vi "addSimulator.vi"(8 "error in (no error)":errorcluster, 10 "IDevice in":refnum<class "IDevice.lvclass">, 11 "IInstance in":refnum<class "IInstance.lvclass">) -> (0 "error out":errorcluster, 2 "IDevice out":refnum<class "IDevice.lvclass">, 3 "IInstance out":refnum<class "IInstance.lvclass">)   [LabVIEW 2022 SP3, in "openDAQ.lvlib" / "daqUtils.lvlib"]
uses:
  daqUtils.lvlib
  IInstance/IInstance.lvclass
  IDevice/IDevice.lvclass
  IDeviceInfo/IDeviceInfo.lvclass
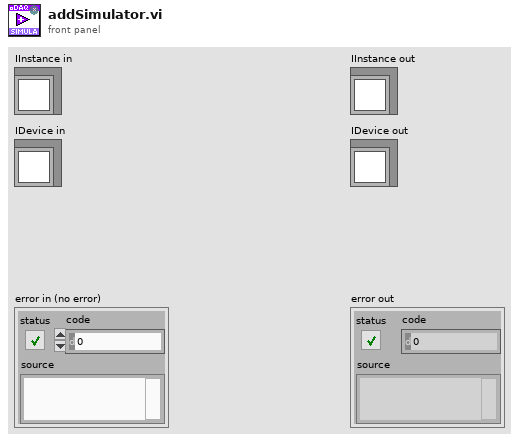
[diagram p1: front panel]
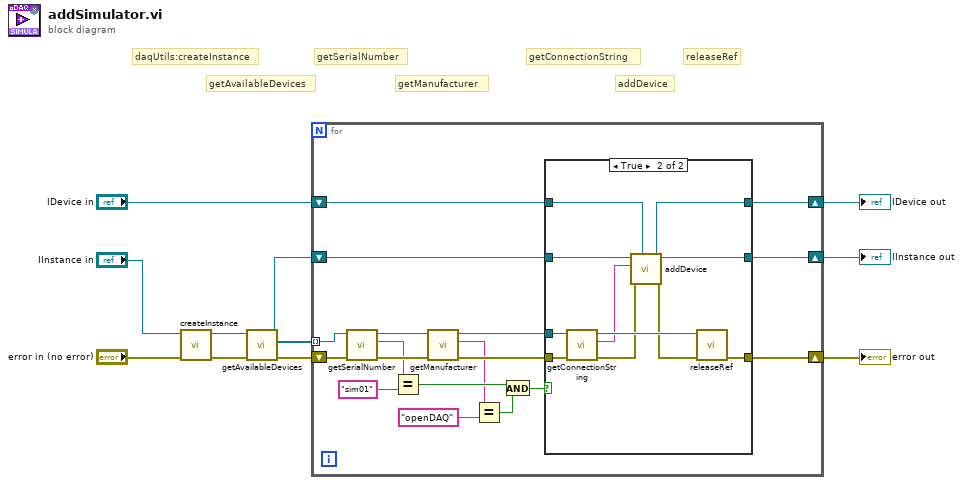
[diagram p0: block diagram]
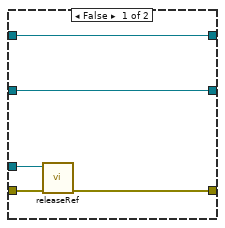
[diagram p2: hidden frame]
diagram:
  # "releaseRef"
  # "addDevice"
  # "getConnectionString"
  # "getManufacturer"
  # "getSerialNumber"
  # "getAvailableDevices"
  # "daqUtils:createInstance"
  n1 = call "createInstance.vi"("error in (no error)"="error in (no error)", "IInstance in"="IInstance in") -> ("error out"=w4:errorcluster, "IInstance out"=w3:refnum<class "IInstance.lvclass">)  [unwired: 8 in]
  n2 = call "getAvailableDevices.vi"("error in (no error)"=w4, "IDevice in"=w3) -> ("error out"=w6:errorcluster, "availableDeviceInfo out"=w5:refnum<class "IDeviceInfo.lvclass">[], "IDevice out"=w7:refnum<class "IInstance.lvclass">)  [unwired: 7 in]
  n3 = for {
    tunnel: w5 -> [w29] mode=indexing
    shift-right: [w20] -> w9
    shift-left: w6 -> [w28]
    shift-right: [w17] -> w10
    shift-left: "IDevice in" -> [w18]
    shift-right: [w16] -> w11
    shift-left: w7 -> [w19]
    n4 = call "getSerialNumber.vi"("error in (no error)"=w28, "IDeviceInfo in"=w29) -> ("error out"=w27:errorcluster, "SerialNumber out"=w15:string, "IDeviceInfo out"=w13:refnum<class "IDeviceInfo.lvclass">)  [unwired: 7 in]
    n5 = Equal?(x=w15, y="sim01") -> (x = y?=w24:bool)
    n6 = call "getManufacturer.vi"("error in (no error)"=w27, "IDeviceInfo in"=w13) -> ("error out"=w21:errorcluster, "Manufacturer out"=w14:string, "IDeviceInfo out"=w12:refnum<class "IDeviceInfo.lvclass">)  [unwired: 7 in]
    n7 = Equal?(x=w14, y="openDAQ") -> (x = y?=w23:bool)
    n8 = And(x=w24, y=w23) -> (x .and. y?=w22:bool)
    n9 = case shown="True" w22 {
      tunnel: w12 -> [w34 w45]
      tunnel: w21 -> [w33 w44]
      tunnel: [w32 w42] -> w20
      tunnel: w19 -> [w30 w41]
      tunnel: w18 -> [w31 w37]
      tunnel: [w31 w35] -> w17
      tunnel: [w30 w36] -> w16
      frame False {
        n10 = call-dynamic "releaseRef.vi"("error in (no error)"=w33, "IBaseObject in"=w34) -> ("error out"=w32:errorcluster)  [unwired: 9 in]
      }
      frame True {
        n11 = call "getConnectionString.vi"("error in (no error)"=w44, "IDeviceInfo in"=w45) -> ("error out"=w40:errorcluster, "ConntectionString out"=w38:string, "IDeviceInfo out"=w43:refnum<class "IDeviceInfo.lvclass">)  [unwired: 7 in]
        n12 = call "addDevice.vi"("ConnectedDevice In"=w37, "error in (no error)"=w40, "ConnectionString in"=w38, "IDevice in"=w41) -> ("error out"=w39:errorcluster, "ConnectedDevice out"=w35:refnum<class "IDevice.lvclass">, "IDevice out"=w36:refnum<class "IInstance.lvclass">)  [unwired: 5 in]
        n13 = call-dynamic "releaseRef.vi"("error in (no error)"=w39, "IBaseObject in"=w43) -> ("error out"=w42:errorcluster)  [unwired: 9 in]
      }
    }
  }
  "IInstance out" <- w11
  "IDevice out" <- w10
  "error out" <- w9
